vi "Router v1.vi"() -> ()   [LabVIEW 2016]
uses:
  Controls/Router - Configuration.ctl
  Controls/Router/Node Block R-W Properties.ctl
  Controls/Router/Block Properties.ctl
  Controls/Router/Router - PXImc Properties.ctl
  Controls/Router/Router - PXImc Card Properties.ctl
  <vilib>/Utility/error.llb/DialogType.ctl
  VIs/Router/Router - Globals.vi
  PXImc Router.lvlib
panel:
  in  "Router Data In":T1={"Master Table Ref"=refnum, "Master Table Size (Bytes)"=0, "Node Properties"=[], "Router - PXImc Properties"={"PXImc Cards Properties"=[{"PXImc Resource Name"="PXI1Slot2", "Reader - PXImc Session Ref"="", "Writer - PXImc Session Ref"="", "Reader Conn ID"=1, "Writer Conn ID"=2}, {"PXImc Resource Name"="PXI1Slot2", "Reader - PXImc Session Ref"="", "Writer - PXImc Session Ref"="", "Reader Conn ID"=3, "Writer Conn ID"=4}], "Connection Timeout (s)"=60.0, "Readers Buffer Size"=25000}}
  in  "stop":bool
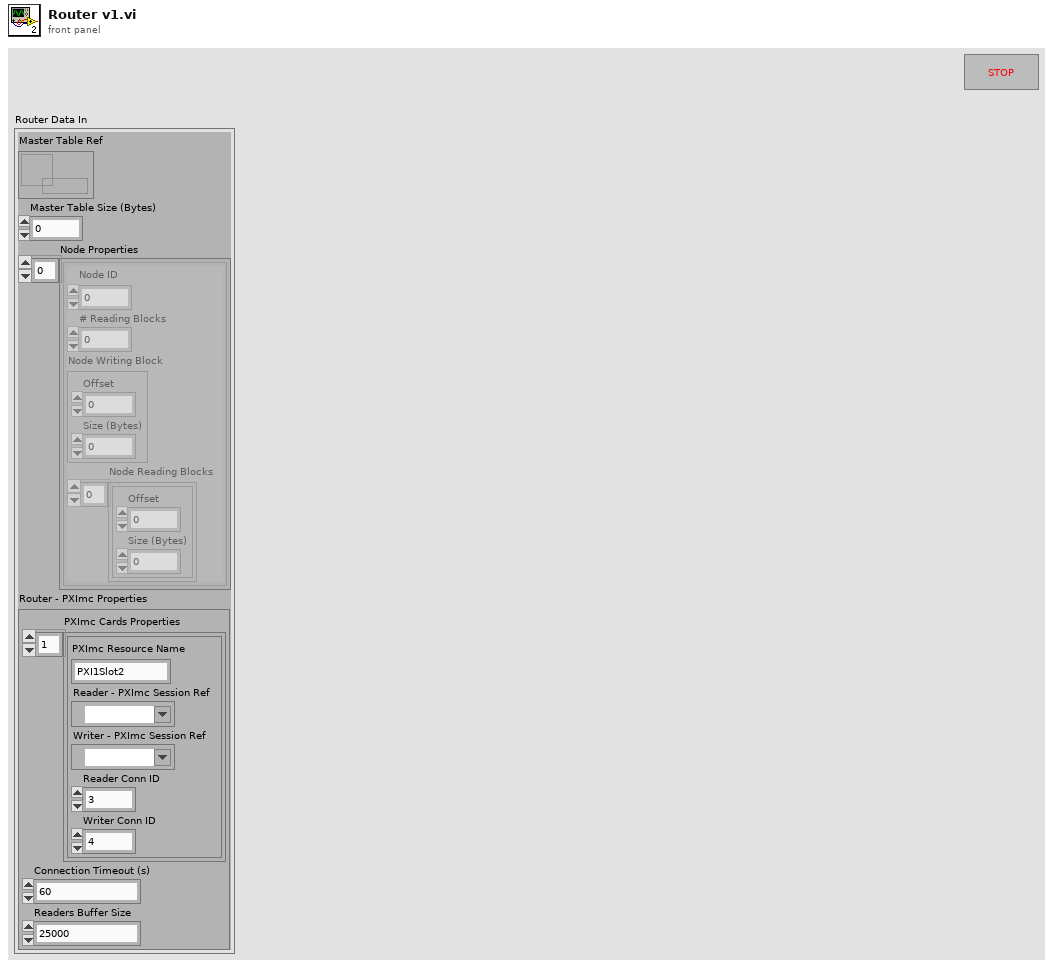
[diagram p1: front panel]
types:
  T1 = typedef "PXImc Router.lvlib/Router - Configuration.ctl" = cluster{"Master Table Ref":refnum<data-value>, "Master Table Size (Bytes)":u32, "Node Properties":T2[], "Router - PXImc Properties":T4}
  T2 = typedef "PXImc Router.lvlib/Node Block R-W Properties.ctl" = cluster{"Node ID":u32, "# Reading Blocks":u32, "Node Writing Block":T3, "Node Reading Blocks":T3[]}
  T3 = typedef "PXImc Router.lvlib/Block Properties.ctl" = cluster{"Offset":u32, "Size (Bytes)":u32}
  T4 = typedef "PXImc Router.lvlib/Router - PXImc Properties.ctl" = cluster{"PXImc Cards Properties":T5[], "Connection Timeout (s)":dbl, "Readers Buffer Size":u64}
  T5 = typedef "PXImc Router.lvlib/Router - PXImc Card Properties.ctl" = cluster{"PXImc Resource Name":string, "Reader - PXImc Session Ref":refnum<k21>, "Writer - PXImc Session Ref":refnum<k21>, "Reader Conn ID":u16, "Writer Conn ID":u16}
  T6 = typedef "DialogType.ctl" = u16
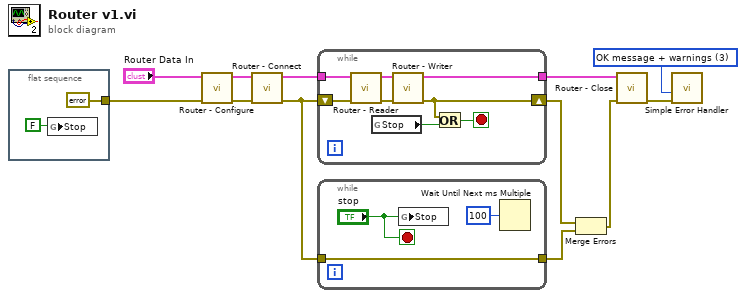
[diagram p0: block diagram]
diagram:
  w11 = T6 3 items=["no dialog", "OK message", "continue or stop message", "OK message + warnings", "continue/stop + warnings"] ("type of dialog (OK msg:1)")
  n1 = flat-sequence {
    tunnel: [errorcluster {"status"=FALSE, "code"=0, "source"=""} ("error constant")] -> w10
    frame #0 {
      n2 = global write "Router - Globals.vi" "Stop"(FALSE ("Stopped")) -> ()
    }
  }
  n3 = call "Router - Configure.vi"("error in (no error)"=w10, "Router Data In"="Router Data In") -> ("error out"=w6:errorcluster, "Router Data Out"=w2:T1)  [unwired: 8 in]
  n4 = call "Router - Connect.vi"("error in (no error)"=w6, "Router Data In"=w2) -> ("error out"=w5:errorcluster, "Router Data Out"=w3:T1)  [unwired: 8 in]
  n5 = while {
    shift-right: [w18] -> w7
    shift-left: w5 -> [w20]
    tunnel: w3 -> [w16]
    tunnel: [w15] -> w1
    stop <- w22 stop-if-true
    n6 = call "Router - Reader.vi"("error in (no error)"=w20, "Router Data In"=w16) -> ("error out"=w19:errorcluster, "Router Data Out"=w17:T1)  [unwired: 8 in]
    n7 = global read "Router - Globals.vi" "Stop"() -> (w21:bool)
    n8 = call "Router - Writer.vi"("error in (no error)"=w19, "Router Data In"=w17) -> ("error out"=w18:errorcluster, "Router Data Out"=w15:T1)  [unwired: 8 in]
    n9 = Or(x=w18, y=w21) -> (x .or. y?=w22:bool)
  }
  n10 = while {
    tunnel: w5 -> [w23]
    tunnel: [w23] -> w9
    stop <- "stop" stop-if-true
    n11 = global write "Router - Globals.vi" "Stop"("stop") -> ()
    n12 = Wait Until Next ms Multiple(millisecond multiple=u32 100) -> ()  [unwired: 1 out]
  }
  n13 = Merge Errors(w7, w9) -> (w8:errorcluster)
  n14 = call "Router - Close.vi"("error in (no error)"=w8, "Router Data In"=w1) -> ("error out"=w12:errorcluster)  [unwired: 9 in]
  n15 = call <vilib>:"Simple Error Handler.vi"("type of dialog (OK msg:1)"=w11, "error in (no error)"=w12) -> ()  [unwired: 3 in, 5 out]
